vi "Enqueue.vi"(8 "Error In":errorcluster, 9 "Data":variant, 10 "Message":string, 11 "queue in":refnum<queue>) -> (0 "Error Out":errorcluster, 3 "queue out":refnum<queue>)   [LabVIEW 2019, in "Queue.lvlib"]
uses:
  Queue.lvlib
  Message Cluster.ctl
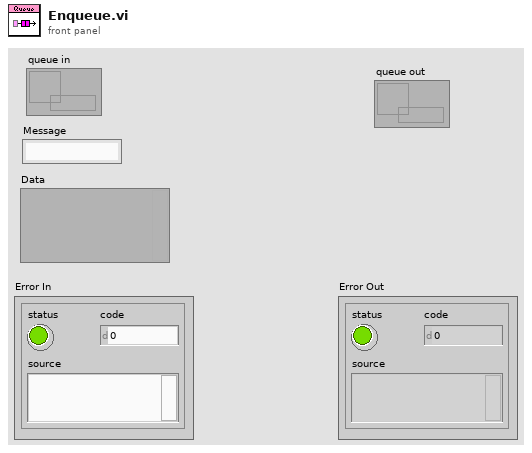
[diagram p1: front panel]
types:
  T1 = typedef "Queue.lvlib/Message Cluster.ctl" = cluster{"Message":string, "Data":variant}
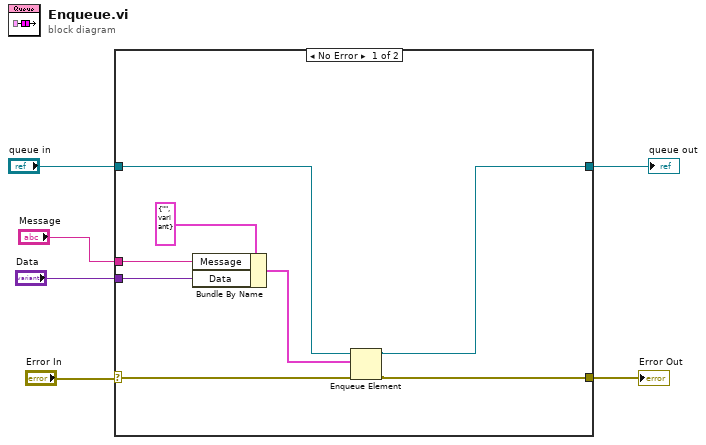
[diagram p0: block diagram]
diagram:
  n1 = case shown="No Error" "Error In" {
    selector: "Error In" -> [w9 w16]
    tunnel: [w7 w16] -> w5
    tunnel: "queue in" -> [w11 w15]
    tunnel: [w8 w15] -> w3
    tunnel: "Message" -> [w13 _]
    tunnel: "Data" -> [w12 _]
    frame No Error {
      n2 = Bundle By Name(cluster=T1 {"Message"="", "Data"=variant} ("element"), "Message"=w13, "Data"=w12) -> (w10:T1)
      n3 = Enqueue Element(queue=w11, element=w10, error in (no error)=w9) -> (queue out=w8:refnum<queue>, error out=w7:errorcluster)  [unwired: 1 in, 1 out]
    }
    frame Error {
    }
  }
  "Error Out" <- w5
  "queue out" <- w3
